vi "WhiteScreenTest_Startup.vi"() -> (0 "ErrorOut":errorcluster)   [LabVIEW 2018] (continued)
-inf, -inf, -inf, -inf, -inf, -inf, -inf, -inf, -inf, -inf, -inf, -inf, -inf, -inf, -inf, -inf, -inf, -inf, -inf, -inf, -inf, -inf, -inf, -inf, -inf, -inf, -inf, -inf, -inf, -inf, -inf, -inf, -inf, -inf, -inf, -inf, -inf, -inf, -inf, -inf, -inf, -inf, -inf, -inf, -inf, -inf, -inf, -inf, -inf, -inf, -inf, -inf, -inf, -inf, -inf, -inf, -inf, -inf, -inf, -inf, -inf, -inf, -inf, -inf, -inf, -inf, -inf, -inf, -inf, -inf, -inf, -inf, -inf, -inf, -inf, -inf, -inf, -inf, -inf, -inf, -inf, -inf, -inf, -inf, -inf, -inf, -inf, -inf, -inf, -inf, -inf, -inf, -inf, -inf, -inf, -inf, -inf, -inf, -inf, -inf, -inf, -inf, -inf, -inf, -inf, -inf, -inf, -inf, -inf, -inf, -inf, -inf, -inf, -inf, -inf, -inf, -inf, -inf, -inf, -inf, -inf, -inf, -inf, -inf, -inf, -inf, -inf, -inf, -inf, -inf, -inf, -inf, -inf, -inf, -inf, -inf, -inf, -inf, -inf, -inf, -inf, -inf, -inf, -inf, -inf, -inf, -inf, -inf, -inf, -inf, -inf, -inf, -inf, -inf, -inf, -inf, -inf, -inf, -inf, -inf, -inf, -inf, -inf, -inf, -inf, -inf, -inf, -inf, -inf, -inf, -inf, -inf, -inf, -inf, -inf, -inf, -inf, -inf, -inf, -inf, -inf, -inf, -inf, -inf, -inf, -inf, -inf, -inf, -inf, -inf, -inf, -inf, -inf, -inf, -inf, -inf, -inf, -inf, -inf, -inf, -inf, -inf, -inf, -inf, -inf, -inf, -inf, -inf, -inf, -inf, -inf, -inf, -inf, -inf, -inf, -inf, -inf, -inf, -inf, -inf, -inf, -inf, -inf, -inf, -inf, -inf, -inf, -inf, -inf, -inf, -inf, -inf, -inf, -inf, -inf, -inf, -inf, -inf, -inf, -inf, -inf, -inf, -inf, -inf, -inf, -inf, -inf, -inf, -inf, -inf, -inf, -inf, -inf, -inf, -inf, -inf, -inf, -inf, -inf, -inf, -inf, -inf, -inf, -inf, -inf, -inf, -inf, -inf, -inf, -inf, -inf, -inf, -inf, -inf, -inf, -inf, -inf, -inf, -inf, -inf, -inf, -inf, -inf, -inf, -inf, -inf, -inf, -inf, -inf, -inf, -inf, -inf, -inf, -inf, -inf, -inf, -inf, -inf, -inf, -inf, -inf, -inf, -inf, -inf, -inf, -inf, -inf, -inf, -inf, -inf, -inf, -inf, -inf, -inf, -inf, -inf, -inf, -inf, -inf, -inf, -inf, -inf, -inf, -inf, -inf, -inf, -inf, -inf, -inf, -inf, -inf, -inf, -inf, -inf, -inf, -inf, -inf, -inf, -inf, -inf, -inf, -inf, -inf, -inf, -inf, -inf, -inf, -inf, -inf, -inf, -inf, -inf, -inf, -inf, -inf, -inf, -inf, -inf, -inf, -inf, -inf, -inf, -inf, -inf, -inf, -inf, -inf, -inf, -inf, -inf, -inf, -inf, -inf, -inf, -inf, -inf, -inf, -inf, -inf, -inf, -inf, -inf, -inf, -inf, -inf, -inf, -inf, -inf, -inf, -inf, -inf, -inf, -inf, -inf, -inf, -inf, -inf, -inf, -inf, -inf, -inf, -inf, -inf, -inf, -inf, -inf, -inf, -inf, -inf, -inf, -inf, -inf, -inf, -inf, -inf, -inf, -inf, -inf, -inf, -inf, -inf, -inf, -inf, -inf, -inf, -inf, -inf, -inf, -inf, -inf, -inf, -inf, -inf, -inf, -inf, -inf, -inf, -inf, -inf, -inf, -inf, -inf, -inf, -inf, -inf, -inf, -inf, -inf, -inf, -inf, -inf, -inf, -inf, -inf, -inf, -inf, -inf, -inf, -inf, -inf, -inf, -inf, -inf, -inf, -inf, -inf, -inf, -inf, -inf, -inf, -inf, -inf, -inf, -inf, -inf, -inf, -inf, -inf, -inf, -inf, -inf, -inf, -inf, -inf, -inf, -inf, -inf, -inf, -inf, -inf, -inf, -inf, -inf, -inf, -inf, -inf, -inf, -inf, -inf, -inf, -inf, -inf, -inf, -inf, -inf, -inf, -inf, -inf, -inf, -inf, -inf, -inf, -inf, -inf, -inf, -inf, -inf, -inf, -inf, -inf, -inf, -inf, -inf, -inf, -inf, -inf, -inf, -inf, -inf, -inf, -inf, -inf, -inf, -inf, -inf, -inf, -inf, -inf, -inf, -inf, -inf, -inf, -inf, -inf, -inf, -inf, -inf, -inf, -inf, -inf, -inf, -inf, -inf, -inf, -inf, -inf, -inf, -inf, -inf, -inf, -inf, -inf, -inf, -inf, -inf, -inf, -inf, -inf, -inf, -inf, -inf, -inf, -inf, -inf, -inf, -inf, -inf, -inf, -inf, -inf, -inf, -inf, -inf, -inf, -inf, -inf, -inf, -inf, -inf, -inf, -inf, -inf, -inf, -inf, -inf, -inf, -inf, -inf, -inf, -inf, -inf, -inf, -inf, -inf, -inf, -inf, -inf, -inf, -inf, -inf, -inf, -inf, -inf, -inf, -inf, -inf, -inf, -inf, -inf, -inf, -inf, -inf, -inf, -inf, -inf, -inf, -inf, -inf, -inf, -inf, -inf, -inf, -inf, -inf, -inf, -inf, -inf, -inf, -inf, -inf, -inf, -inf, -inf, -inf, -inf, -inf, -inf, -inf, -inf, -inf, -inf, -inf, -inf, -inf, -inf, -inf, -inf, -inf, -inf, -inf, -inf, -inf, -inf, -inf, -inf, -inf, -inf, -inf, -inf, -inf, -inf, -inf, -inf, -inf, -inf, -inf, -inf, -inf, -inf, -inf, -inf, -inf, -inf, -inf, -inf, -inf, -inf, -inf, -inf, -inf, -inf, -inf, -inf, -inf, -inf, -inf, -inf, -inf, -inf, -inf, -inf, -inf, -inf, -inf, -inf, -inf, -inf, -inf, -inf, -inf, -inf, -inf, -inf, -inf, -inf, -inf, -inf, -inf, -inf, -inf, -inf, -inf, -inf, -inf, -inf, -inf, -inf, -inf, -inf, -inf, -inf, -inf, -inf, -inf, -inf, -inf, -inf, -inf, -inf, -inf, -inf, -inf, -inf, -inf, -inf, -inf, -inf, -inf, -inf, -inf, -inf, -inf, -inf, -inf, -inf, -inf, -inf, -inf, -inf, -inf, -inf, -inf, -inf, -inf, -inf, -inf, -inf, -inf]
  out "df (Hz)":dbl=15258.7890625
  in  "AutoScale Y Noise":bool caption="AutoScale Y"
  in  "AvgAvg":bool caption="Average over 1 minute"
  out "Power History 84 X":T13(graph)
  out "Power History 84 Co":T13(graph)
  out "Power History 72 X":T13(graph)
  out "Power History 72 Co":T13(graph)
  in  "NewValueWeighting":dbl=0.75 min=0.01 max=1.0 step=0.01
  out "Freq History 84 Co":cluster{dbl, dbl, dbl}(graph)
  out "Freq History 84 X":cluster{dbl, dbl, dbl}(graph)
  out "Freq History 72 X":cluster{dbl, dbl, dbl}(graph)
  out "Freq History 72 Co":cluster{dbl, dbl, dbl}(graph)
  out "Inclinometer Std Dev History":T14(graph)
  out "Inclinometer History":T14(graph)
  out "VoltageDisplay":T15={"AI0_Unused"=0.033825768742891164, "AI1_-5V"=0.03350358521901454, "AI2_+5V"=0.03414795226674084, "AI3_+6V"=-0.0003256849402108635, "AI4_+12V"=-0.0012922355206829907, "AI5_+15V"=-0.0012922355206829907, "AI6_+28V"=-0.020301063655153495, "Ai16_72GHz_CalPower"=-0.0022587861014084333, "Ai17_84GHz_CalPower"=-0.0038697037365145624, "Ai18_InclinometerAz"=-0.0038697037365145624, "Ai19_InclinometerEl"=-0.0038697037365145624, "Az_StdDev"=-0.0038697037365145624, "El_StdDev"=-0.0038697037365145624, "Ai20_BlowerPower"=-0.0038697037365145624} caption="Voltage" {"Ai20_BlowerPower" format="%#.2g"; "El_StdDev" format="%#.2g"; "Az_StdDev" format="%#.2g"; "Ai19_InclinometerEl" format="%#.2g"; "Ai18_InclinometerAz" format="%#.2g"; "Ai17_84GHz_CalPower" format="%#.4g"; "Ai16_72GHz_CalPower" format="%#.4g"; "AI6_+28V" format="%#.2g"; "AI5_+15V" format="%#.2g"; "AI4_+12V" format="%#.2g"; "AI3_+6V" format="%#.2g"; "AI2_+5V" format="%#.2g"; "AI1_-5V" format="%#.2g"; "AI0_Unused" format="%#.2g"}
  out "TCsDisplay":T16={"TC0_LP1_Hi"=25.446637506096643, "TC1_LP1_MidHi"=-67954.67080824148, "TC2_LP1_Mid"=-67954.0860092046, "TC3_LP1_LoMid"=-68014.21654976695, "TC4_LP1_Lo"=-68013.6313297234, "TC5_LP2_Hi"=-68014.21654976695, "TC6_LP2_MidHi"=-68058.43020070596, "TC7_LP2_Mid"=-68059.01573745323, "TC8_LP2_LoMid"=-67937.01745222262, "TC9_LP2_Lo"=-67937.60213056742, "TC10_HVAC_Cond_In"=-67937.01745222262, "TC11_HVAC_Cond_Out"=-68021.98391844248, "TC12_Gen_Exhaust"=-68021.39864348577, "TC13_Tamb_Interior"=-68021.39864348577} caption="Thermocouples" {"TC13_Tamb_Interior" format="%#.1f"; "TC12_Gen_Exhaust" format="%#.1f"; "TC11_HVAC_Cond_Out" format="%#.1f"; "TC10_HVAC_Cond_In" format="%#.1f"; "TC9_LP2_Lo" format="%#.1f"; "TC8_LP2_LoMid" format="%#.1f"; "TC7_LP2_Mid" format="%#.1f"; "TC6_LP2_MidHi" format="%#.1f"; "TC5_LP2_Hi" format="%#.1f"; "TC4_LP1_Lo" format="%#.1f"; "TC3_LP1_LoMid" format="%#.1f"; "TC2_LP1_Mid" format="%#.1f"; "TC1_LP1_MidHi" format="%#.1f"; "TC0_LP1_Hi" format="%#.1f"}
  out "84CoCalFrq":dbl format="%#.9f"
  out "MaxValue_Cal_84X":dbl format="%#.2g"
  out "84CoBeacFrq":dbl format="%#.9f"
  out "MaxValue_Cal_72X":dbl format="%#.2g"
  out "72CoCalFrq":dbl format="%#.9f"
  out "72CoBeacFrq":dbl format="%#.2f"
  out "ADAM-Noise":dbl format="%#.2g"
  out "ADAM-CalEncl":dbl format="%#.2g"
  out "ADAM-XPol":dbl format="%#.2g"
  out "ADAM-Co":dbl format="%#.2g"
  out "TE_Front":dbl format="%#.2g"
  out "TE_Bottom":dbl format="%#.2g"
  out "TE_Air":dbl format="%#.2g"
  out "InclEl":dbl format="%#.2g"
  out "InclAz":dbl format="%#.2g"
  out "MaxValue_Cal_84Co":dbl format="%#.2g"
  out "MaxValue_Cal_72Co":dbl format="%#.2g"
  out "+28":dbl format="%#.2g"
  out "+15":dbl format="%#.2g"
  out "+12":dbl format="%#.2g"
  out "+6":dbl format="%#.2g"
  out "+5":dbl format="%#.2g"
  out "-5V":dbl format="%#.2g"
  out "ConnextIntTemp":dbl format="%#.2g"
  in  "AlarmThresholds_OneChan":T17={"Enbl"=FALSE, "ErrsAndWarns"={2.256637168141593, 5.663716814159292, 7.168141592920354, 9.336283185840708}} {"ErrsAndWarns" scale=0.0..10.0}
  in  "AlarmSettings":T18={"TC13"={"Enbl"=FALSE, "ErrsAndWarns"={0.0, 5.663716814159292, 7.168141592920354, 8.584070796460177}}, "AI1"={"Enbl"=FALSE, "ErrsAndWarns"={0.0, 5.663716814159292, 7.168141592920354, 8.584070796460177}}, "AI2"={"Enbl"=FALSE, "ErrsAndWarns"={0.0, 5.663716814159292, 7.168141592920354, 8.584070796460177}}, "AI3"={"Enbl"=FALSE, "ErrsAndWarns"={0.0, 5.663716814159292, 7.168141592920354, 8.584070796460177}}, "AI4"={"Enbl"=FALSE, "ErrsAndWarns"={0.0, 5.663716814159292, 7.168141592920354, 8.584070796460177}}, "AI5"={"Enbl"=FALSE, "ErrsAndWarns"={0.0, 5.663716814159292, 7.168141592920354, 8.584070796460177}}, "AI6"={"Enbl"=FALSE, "ErrsAndWarns"={0.0, 5.663716814159292, 7.168141592920354, 8.584070796460177}}, "AI18"={"Enbl"=FALSE, "ErrsAndWarns"={0.0, 5.663716814159292, 7.168141592920354, 8.584070796460177}}, "AI19"={"Enbl"=FALSE, "ErrsAndWarns"={0.0, 5.663716814159292, 7.168141592920354, 8.584070796460177}}, "TE1"={"Enbl"=FALSE, "ErrsAndWarns"={0.0, 5.663716814159292, 7.168141592920354, 8.584070796460177}}, "TE2"={"Enbl"=TRUE, "ErrsAndWarns"={0.0, 5.663716814159292, 7.168141592920354, 8.584070796460177}}, "TE3"={"Enbl"=FALSE, "ErrsAndWarns"={0.0, 5.663716814159292, 7.168141592920354, 8.584070796460177}}, "ADAM1"={"Enbl"=FALSE, "ErrsAndWarns"={0.0, 5.663716814159292, 7.168141592920354, 8.584070796460177}}, "ADAM2"={"Enbl"=FALSE, "ErrsAndWarns"={0.0, 5.663716814159292, 7.168141592920354, 8.584070796460177}}, "ADAM3"={"Enbl"=FALSE, "ErrsAndWarns"={0.0, 5.663716814159292, 7.168141592920354, 8.584070796460177}}, "ADAM4"={"Enbl"=FALSE, "ErrsAndWarns"={0.0, 5.663716814159292, 7.168141592920354, 8.584070796460177}}, "72CoBeacFreq"={"Enbl"=FALSE, "ErrsAndWarns"={0.0, 5.663716814159292, 7.168141592920354, 8.584070796460177}}, "72CoCalFreq"={"Enbl"=FALSE, "ErrsAndWarns"={0.0, 5.663716814159292, 7.168141592920354, 8.584070796460177}}, "84CoBeacFreq"={"Enbl"=FALSE, "ErrsAndWarns"={0.0, 5.663716814159292, 7.168141592920354, 8.584070796460177}}, "84CoCalFreq"={"Enbl"=FALSE, "ErrsAndWarns"={0.0, 5.663716814159292, 7.168141592920354, 8.584070796460177}}, "72Co_CalTonePwr"={"Enbl"=FALSE, "ErrsAndWarns"={-110.0, -90.0, -65.0, -60.0}}, "72X_CalTonePwr"={"Enbl"=FALSE, "ErrsAndWarns"={0.0, 5.663716814159292, 7.168141592920354, 8.584070796460177}}, "84Co_CalTonePwr"={"Enbl"=FALSE, "ErrsAndWarns"={0.0, 5.663716814159292, 7.168141592920354, 8.584070796460177}}, "84X_CalTonePwr"={"Enbl"=FALSE, "ErrsAndWarns"={0.0, 5.663716814159292, 7.168141592920354, 8.584070796460177}}} {"84X_CalTonePwr"."ErrsAndWarns" scale=-120.0..-55.0; "72X_CalTonePwr"."ErrsAndWarns" scale=-120.0..-55.0; "84Co_CalTonePwr"."ErrsAndWarns" scale=-120.0..-55.0; "72Co_CalTonePwr"."ErrsAndWarns" scale=-120.0..-55.0; "84CoCalFreq"."ErrsAndWarns" scale=24.9..25.1; "84CoBeacFreq"."ErrsAndWarns" scale=25.3..25.8; "72CoCalFreq"."ErrsAndWarns" scale=24.9..25.1; "72CoBeacFreq"."ErrsAndWarns" scale=25.4..25.8; "ADAM4"."ErrsAndWarns" scale=30.0..52.0; "ADAM3"."ErrsAndWarns" scale=30.0..52.0; "ADAM2"."ErrsAndWarns" scale=30.0..52.0; "ADAM1"."ErrsAndWarns" scale=30.0..52.0; "TE3"."ErrsAndWarns" scale=30.0..52.0; "TE2"."ErrsAndWarns" scale=30.0..52.0; "TE1"."ErrsAndWarns" scale=20.0..52.0; "AI19"."ErrsAndWarns" scale=0.0..6.0; "AI18"."ErrsAndWarns" scale=0.0..8.0; "AI6"."ErrsAndWarns" scale=0.0..35.0; "AI5"."ErrsAndWarns" scale=0.0..20.0; "AI4"."ErrsAndWarns" scale=0.0..15.0; "AI3"."ErrsAndWarns" scale=0.0..10.0; "AI2"."ErrsAndWarns" scale=0.0..10.0; "TC13"."ErrsAndWarns" scale=0.0..40.0}
  out "Elapsed_SNR_Timer":dbl caption="Elapsed SNR Timer"
  in  "Trouble Shooting Tabs":T19(tab)
  out "Q Probes":T20
  out "Probe 21":fxp<+/-,24,5>=-4.57763671875e-05
  out "Probe 22":fxp<+/-,54,35>=-15871.999969482422
  out "Probe 23":fxp<+/-,54,1>=-7.629394517039145e-06
  out "Probe 24":fxp<+/-,16,1>
  out "I Probes":T20
  out "Probe 3":fxp<+/-,39,24>=-0.003662109375
  out "Probe 1":i16=-27
  out "Probe 2":fxp<+/-,16,16>
  out "Probe 5":fxp<+/-,16,2>
  out "Probe 7":fxp<+/-,18,1>
  out "ReceiverTimed Out":bool
  out "NoiseFloorFIFOTimeOut":bool
  out "Probe Offsetd":fxp<+/-,16,16>
  in  "Target to Probe":T21=enum."4"
  in  "Time Domain Tabs":T22(tab)
  out "TimeDomainCal":ext[](graph)
  out "TimeDomainBeac":ext[](graph)
  out "TimeDomainCal 2":ext[](graph)
  out "TimeDomainBeacon 2":ext[](graph)
  out "TimeDomainCal 3":ext[](graph)
  out "TimeDomain Beac 3":ext[](graph)
  out "InPhase Spect":dbl[](graph)
  out "QuadratureSpect":dbl[](graph)
  out "TimeDomainCal 4":ext[](graph)
  out "TimeDomainBeacon 4":ext[](graph)
  out "Memory Used":dbl(graph)=797012.0
  out "CalShift 2":dbl=24999500.0 format="%#_10g"
  out "BeaconShift 2":dbl=26246000.0 format="%#_10g"
  out "BeaconShift":dbl=26246000.0 format="%#_10g"
  out "CalShift":dbl=24999500.0 format="%#_10g"
  out "FAM Initialized?":bool=TRUE
  out "Memory Used By LV (KB)":dbl=797012.0
  out "BeaconShift 4":dbl=26244800.0 format="%#_10g"
  out "BeaconShift 3":dbl=26246000.0 format="%#_10g"
  out "CalShift 3":dbl=24999500.0 format="%#_10g"
  out "CalShift 4":dbl=24998000.0 format="%#_10g"
  in  "MemoryPlotRate":dbl=30.0 format="%#_13g"
  out "SPVSR_Count":i32
  out "SPVSR_Queue":i32
  out "FP_Count":i32
  out "# in FP queue":i32
  out "PhaseCount 1":u64
  out "PhaseCount 2":u64
  out "PhaseCount 3":u64
  out "PhaseCount 4":u64
  out "X I_Index":ext[](array[numeric])
  out "72 Co Beac Q":ext[](graph)
  out "72 Co Beac I":ext[](graph)
  out "Co I_Index":ext[](array[numeric])
  in  "Exit":bool
  in  "Stop":bool
  # "Ugh5"
  # "Copyright © 2020 Epimedia, Inc. All Rights Reserved.\n\nThe Epimedia Application Library is Copyright © 2009-2020 Epimedia, Inc. \nAll Rights Reserved. Used under license."
  # "Angle_out = [(V_reading – Vmin) / Vmax ) * (Angle_max - Angle_min) + Angle_min + Angle_offset ] * (-1 if pos_neg toggle switch is on)\n\nThe default (equivalent to current equation) values would be\nVmin = 0\nVmax = 4.5\nAngle_min = -90\nAngle_range = Angle_max-Angle_min\nAngle_max = 90\nAngle_offset = 0\nPos_neg = off"
  # "72 Cross Tracking Frequency is linked to 72 Co"
  # "84 Cross Tracking Frequency is linked to 84 Co"
  # "72 Co"
  # "84 Co"
  # "72 GHz"
  # "84 GHz"
  # "Enable/disable"
  # "The digital readouts display the same errors and \nwarnings with more precision."
  # "Low Error"
  # "Low Warning"
  # "High Warning"
  # "High Error"
  # "seconds"
  # "I Probes"
  # "Q Probes"
  # "-1 to 0.999, d:7.629e-6"
  # "Shifted"
  # "I16"
  # "-1 to 1, d:1.92e-7"
  # "From digitizer"
  # "Filtered Step 4"
  # "-3.27e4 to 3.27e4, d:1"
  # "-1 to 1, d:1.92e-7"
  # "To FXP"
  # "Scaled and reduced data size"
  # "-3.27e4 to 3.27e4, d:1"
  # "-1 to 1, d:1.92e-7"
  # "Filtered Step 5"
  # "-6.55e4 to 6.55e4, d:3.05e-5"
  # "-8.39e6 to 8.39e6, d:1.19e-7"
  # "Scaled"
  # "Scaled after Step 5"
  # "XXX"
  # "-2 to 2, d:2.38e-7"
  # "-2 to 1.999, d:6.10e-5"
  # "Filtered Step 6"
  # "Filtered stage A"
  # "-1.677e7 to 1.677e7, d:2.38e-7"
  # "Scaled after Step 6"
  # "XXX"
  # "-2.62e5 to 2.62e5, d:6.10e-5"
  # "Scaled (Step 1 Scale)"
  # "-1 to 1, d:1.82e-12"
  # "Filtered Step 7"
  # "-8.39e6 to 8.39e6, d:1.82e-12"
  # "Filtered after Step 7"
  # "XXX"
  # "-8.39e6 to 8.39e6, d:1.82e-12"
  # "Sent to host\nIdentical to 18"
  # "Noise Floor"
  # "-4 to 4"
  # "-3.35e7 to 3.35e7, d:4.7e-7"
  # "-1 to 1, d:1.4e-14"
  # "-1 to .99, d:3.05e-5"
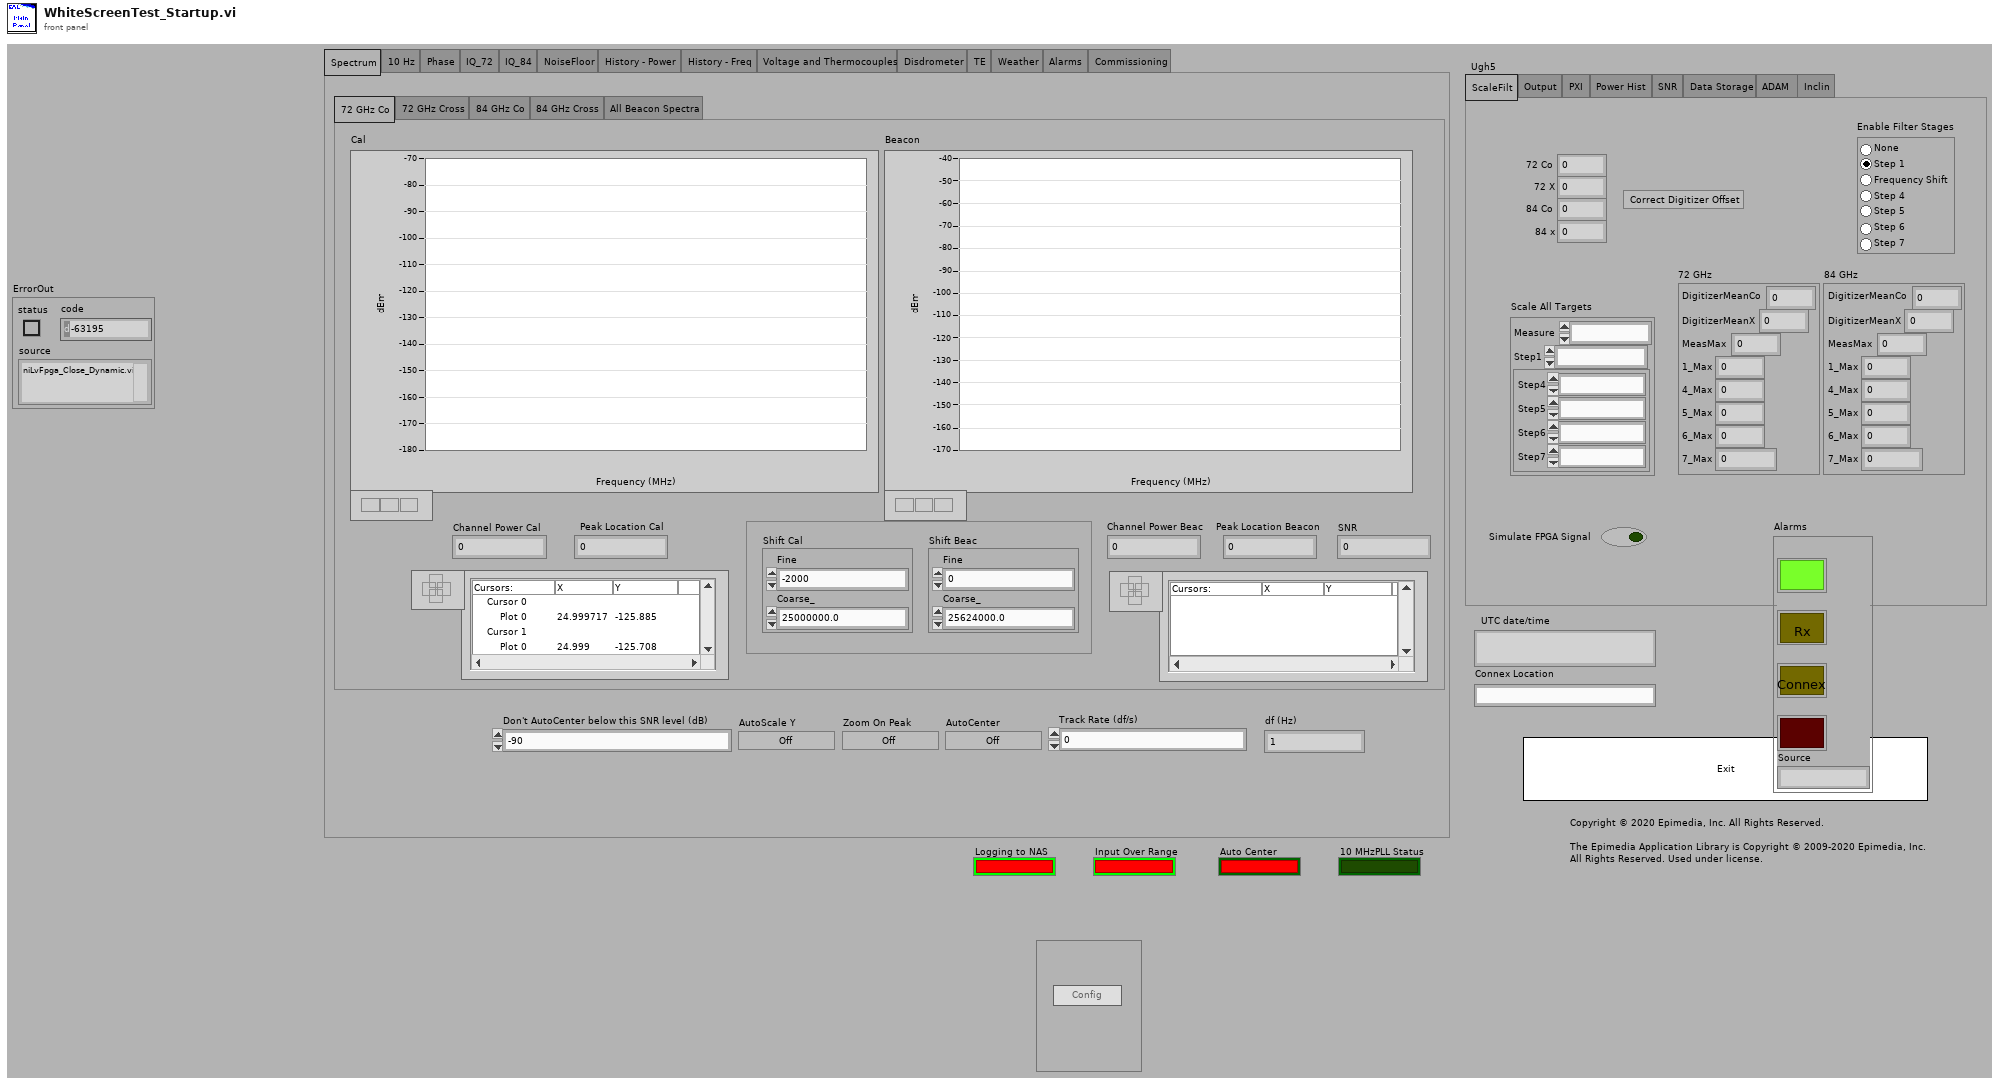
[diagram p1: front panel]
types:
  T1 = typedef "DigOutClust.ctl" = cluster{"Green":bool, "Rx_Yell":bool, "Cx_Yell":bool, "Red":bool, "Source":string}
  T2 = enum32{"ScaleFilt", "Output", "PXI", "Power Hist", "SNR", "Data Storage", "ADAM", "Inclin"}
  T3 = typedef "SaturationMonitor.ctl" = cluster{"MeasMean0":dbl, "MeasMean1":dbl, "MeasMax":dbl, "1_Max":dbl, "4_Max":dbl, "5_Max":dbl, "6_Max":dbl, "7_Max":dbl}
  T4 = typedef "ScaleTargetClust.ctl" = cluster{"Measure":fxp<+/-,16,1>, "Step1":fxp<+/-,17,17>, "Scale":T5}
  T5 = typedef "FPGA_Scale.ctl" = cluster{"Step4":fxp<+/-,23,23>, "Step5":fxp<+/-,23,23>, "Step6":fxp<+/-,23,23>, "Step7":fxp<+/-,23,23>}
  T6 = typedef "FilterEnableRadio.ctl" = enum32{"None", "Step 1", "Frequency Shift", "Step 4", "Step 5", "Step 6", "Step 7"}
  T7 = cluster{"Cal Smooth":dbl, "Beac Smooth":dbl, "Cal Smooth":dbl, "Beac Smooth":dbl, "Cal Smooth":dbl, "Beac Smooth":dbl, "Cal Smooth":dbl, "Beac Smooth":dbl}
  T8 = typedef "Inclinometer_User_Cfg.ctl" = cluster{"Vmin":dbl, "Vmax":dbl, "Angle_min":dbl, "Angle_max":dbl, "Offset":dbl, "Pos_Neg":bool}
  T9 = enum32{"Spectrum", "10 Hz", "Phase", "IQ_72", "IQ_84", "NoiseFloor", "History - Power", "History - Freq", "Voltage and Thermocouples", "Disdrometer", "TE", "Weather", "Alarms", "Commissioning"}
  T10 = enum32{"72 GHz Co", "72 GHz Cross", "84 GHz Co", "84 GHz Cross", "All Beacon Spectra"}
  T11 = typedef "FreqShift.ctl" = cluster{"Fine":dbl, "Coarse_":dbl}
  T12 = enum32{"72 GHz Co", "72 GHz Cross", "84 GHz Co", "84 GHz Cross"}
  T13 = cluster{"Cal":dbl, "Cal Smooth":dbl, "Beac":dbl, "Beac Smooth":dbl, "NoiseFloorSum":dbl, "NoiseFloorSum Smooth":dbl}
  T14 = cluster{"Ai18_InclinometerAz":dbl, "Ai19_InclinometerEl":dbl}
  T15 = typedef "Voltage_Display_Clust.ctl" = cluster{"AI0_Unused":dbl, "AI1_-5V":dbl, "AI2_+5V":dbl, "AI3_+6V":dbl, "AI4_+12V":dbl, "AI5_+15V":dbl, "AI6_+28V":dbl, "Ai16_72GHz_CalPower":dbl, "Ai17_84GHz_CalPower":dbl, "Ai18_InclinometerAz":dbl, "Ai19_InclinometerEl":dbl, "Az_StdDev":dbl, "El_StdDev":dbl, "Ai20_BlowerPower":dbl}
  T16 = typedef "TC_Display_Clust.ctl" = cluster{"TC0_LP1_Hi":dbl, "TC1_LP1_MidHi":dbl, "TC2_LP1_Mid":dbl, "TC3_LP1_LoMid":dbl, "TC4_LP1_Lo":dbl, "TC5_LP2_Hi":dbl, "TC6_LP2_MidHi":dbl, "TC7_LP2_Mid":dbl, "TC8_LP2_LoMid":dbl, "TC9_LP2_Lo":dbl, "TC10_HVAC_Cond_In":dbl, "TC11_HVAC_Cond_Out":dbl, "TC12_Gen_Exhaust":dbl, "TC13_Tamb_Interior":dbl}
  T17 = typedef "AlarmThresh_OneChan.ctl" = cluster{"Enbl":bool, "ErrsAndWarns":cluster{dbl, dbl, dbl, dbl}}
  T18 = typedef "AlarmSettingsClust.ctl" = cluster{"TC13":T17, "AI1":T17, "AI2":T17, "AI3":T17, "AI4":T17, "AI5":T17, "AI6":T17, "AI18":T17, "AI19":T17, "TE1":T17, "TE2":T17, "TE3":T17, "ADAM1":T17, "ADAM2":T17, "ADAM3":T17, "ADAM4":T17, "72CoBeacFreq":T17, "72CoCalFreq":T17, "84CoBeacFreq":T17, "84CoCalFreq":T17, "72Co_CalTonePwr":T17, "72X_CalTonePwr":T17, "84Co_CalTonePwr":T17, "84X_CalTonePwr":T17}
  T19 = enum32{"FPGA Probes", "Time Domain", "Win Probes", "DeltaPhaseTest"}
  T20 = cluster{"Probe 8":fxp<+/-,18,1>, "Probe 9":fxp<+/-,24,1>, "Probe 10":fxp<+/-,24,1>, "Probe 11":fxp<+/-,24,1>, "Probe 12":fxp<+/-,47,24>, "Probe 13":fxp<+/-,24,1>, "Probe 14":fxp<+/-,25,2>, "Probe 15":fxp<+/-,48,25>, "Probe 16":fxp<+/-,24,1>, "Probe 17":fxp<+/-,25,2>, "Probe 18":fxp<+/-,48,25>, "Probe 19":fxp<+/-,24,1>, "Probe20":fxp<+/-,24,1>}
  T21 = typedef "TargetNumber.ctl" = enum16{"1", "2", "3", "4"}
  T22 = enum32{"Target 1", "Target 2", "Target 3", "Complex Spectra", "Target 4"}
  T23 = typedef "10Hz_Loop_Enum.ctl" = enum16{"10Hz_Init", "10Hz_Cfg", "10Hz_NewData", "10Hz_Write", "10Hz_Stop"}
  T24 = typedef "FP_Loop_Clust.ctl" = cluster{"Alarms":T1, "Spectrum 1":dbl[], "Spectrum 2":dbl[], "Spectrum 3":dbl[], "Spectrum 4":dbl[], "HistoryWeighting":dbl, "NoiseFloorSums":T25, "PwrHist":T26}
  T25 = typedef "NoiseFLoorSums.ctl" = cluster{"1":dbl, "2":dbl, "3":dbl, "4":dbl}
  T26 = typedef "PowerHistory_All.ctl" = cluster{"72Co":cluster{"Cal":dbl, "Cal Smooth":dbl, "Beac":dbl, "Beac Smooth":dbl, "NoiseFloorSum":dbl, "NoiseFloorSum Smooth":dbl}, "72X":cluster{"Cal":dbl, "Cal Smooth":dbl, "Beac":dbl, "Beac Smooth":dbl, "NoiseFloorSum":dbl, "NoiseFloorSum Smooth":dbl}, "84Co":cluster{"Cal":dbl, "Cal Smooth":dbl, "Beac":dbl, "Beac Smooth":dbl, "NoiseFloorSum":dbl, "NoiseFloorSum Smooth":dbl}, "84X":cluster{"Cal":dbl, "Cal Smooth":dbl, "Beac":dbl, "Beac Smooth":dbl, "NoiseFloorSum":dbl, "NoiseFloorSum Smooth":dbl}}
  T27 = typedef "HWQueueElements.ctl" = enum16{"HW_Init", "HW_UpdtCfg", "HW_Start", "HW_Pause", "HW_Run", "HW_Cls", "HW_Exit"}
  T28 = typedef "FP_Loop_Enum.ctl" = enum16{"FP_Init", "FP_Scale", "FP_Tone", "FP_Noise", "FP_Probes", "FP_PXI", "FP_AI", "FP_TC", "FP_PWR_Hist", "FP_Alarm", "FP_Exit"}
  T29 = typedef "DigiLoopEnum.ctl" = enum16{"Dig_Init", "Digi_Write", "Digi_Exit"}
  T30 = typedef "LogLoopEnum.ctl" = enum16{"Log_Init", "Log_Config", "Log_CfgAlarm", "Log_TimeDomain", "Log_Tone", "Log_NoiseTrace", "Log_NoiseSum", "Log_DO", "Log_AI", "Log_TC", "Log_Disdrom", "Log_Weather", "Log_TE", "Log_ADAM", "Log_UPS", "Log_ChkTime", "Log_Alarm", "Log_Write", "Log_Exit"}
  T31 = typedef "NoiseQueueElements.ctl" = enum16{"Noise_Startup", "Noise_Init", "Noise_Macro", "Noise_Config", "Noise_NewData", "Noise_Transform", "Noise_SumdTrace", "Noise_Send", "Noise_Probes", "Noise_Exit"}
  T32 = typedef "MasterCluster.ctl" = cluster{"Admin":T33, "RTConfig":T35, "SMS":T36, "FPGA":T37, "Config":T38, "Stat":T44, "Alarm":T18}
  T33 = typedef "AdminCluster.ctl" = cluster{"Lvl":T34, "Pwd":string}
  T34 = typedef "UserLevelEnum.ctl" = enum16{"Admin", "Operator"}
  T35 = typedef "RT_Config.ctl" = cluster{"Arm":bool, "Number":dbl, "String":string}
  T36 = typedef "SMSDataCluster.ctl" = cluster{"Enbl?":bool, "Addr":string[]}
  T37 = typedef "FPGA_Config_Clust.ctl" = cluster{"Target":T21, "Channel":T21, "Ref1":refnum<k20>, "Ref2":refnum<k20>}
  T38 = typedef "Config_Clust.ctl" = cluster{"UsrCfg":T39, "FP_User":T41}
  T39 = typedef "UserConfig.ctl" = cluster{"Paths":T40, "SampleRate":dbl}
  T40 = typedef "PathsCluster.ctl" = cluster{"CfgFile":path, "LogFolder":path, "LogFile":path, "NAS path":path, "ThreshFile":path, "RedunFolder":path}
  T41 = typedef "FrontPanel_UserConfig.ctl" = cluster{"#NoiseSums":u32, "Max_df":u32, "AvgAvg":bool, "#Avg":u16, "AutoCenter":bool, "Inclin":T8, "1":T42, "2":T42, "3":T42, "4":T42, "Target to Probe":T21, "SNR_Thresh":dbl, "Paths":T40, "Connex_Location":string, "SimulateFPGA":bool}
  T42 = typedef "FP_UserTargetConfig.ctl" = cluster{"Cal_":T11, "Beac":T11, "Scale":T5, "Offset":fxp<+/-,16,16>, "Scale_Noise":fxp<+/-,30,30>, "Scale_Step1":fxp<+/-,17,17>, "Scale_In_RT":ext, "ScaleMeas":fxp<+/-,16,1>, "FreqsToRemove":i32[], "Width":i32[], "ScaleMeasEnum":T43, "FilterEnab":T6}
  T43 = typedef "ScaleMeasure.ctl" = enum16{"1", "10", "50", "42"}
  T44 = typedef "SystemStatusCluster.ctl" = cluster{"SysState":T45, "TrackRate":bool, "AutoCentr":bool}
  T45 = typedef "SystemStateEnum.ctl" = enum16{"Init", "Idle", "Running", "System Fault", "System Error", "Exit"}
  T46 = typedef "DataQueueElements.ctl" = enum16{"Data_Init", "Data_Config", "Data_AddData", "Data_FreqShift", "Data_FPGA_Write", "Data_Transform", "Data_Send", "Data_Exit"}
  T47 = typedef "MainQueueElements.ctl" = enum16{"Spvsr_InitQ", "Spvsr_RfrshPnl", "Spvsr_InitSW", "Spvsr_InitCtrls", "Spvsr_Cursors", "Spvsr_StrtHWLp", "Spvsr_Stop", "Spvsr_NewData", "Spvsr_ScaleGraphs", "Spvsr_Error", "Spvsr_About", "Spvsr_Config", "Spvsr_FPConfig", "Spvsr_AlarmCfg", "Spvsr_DigitzOffs", "FP_AO_ctrl", "Spvsr_RestartWarn", "Spvsr_AutoCenter", "Spvsr_TrackRate", "Spvsr_ChkTime", "Spvsr_Admin", "Spvsr_Exit"}
  T48 = typedef "HDF5_10HzRefs.ctl" = cluster{"72Co_dset":T49, "84Co_dset":T49, "FileRef":T49}
  T49 = typedef "hid_t.ctl" = i32
  T50 = typedef "AI_Type_Enum.ctl" = enum16{"AI", "TC"}
  T51 = typedef "MainQueueElements.ctl" = enum16{"Spvsr_InitQ", "Spvsr_RfrshPnl", "Spvsr_InitSW", "Spvsr_InitCtrls", "Spvsr_Cursors", "Spvsr_StrtHWLp", "Spvsr_Stop", "Spvsr_NewData", "Spvsr_DigiOut", "Spvsr_ScaleGraphs", "Spvsr_Error", "Spvsr_About", "Spvsr_Config", "Spvsr_FPConfig", "Spvsr_AlarmCfg", "Spvsr_DigitzOffs", "FP_AO_ctrl", "Spvsr_RestartWarn", "Spvsr_AutoCenter", "Spvsr_TrackRate", "Spvsr_ChkTime", "Spvsr_Admin", "Spvsr_Exit"}
  T52 = enum8{"Enabled", "Disabled", "Disabled and Grayed Out"}
  T53 = typedef "AI_Loop_Enum.ctl" = enum16{"AI_Init", "AI_Config", "AI_Alarm", "AI_Read", "AI_ChkTime", "AI_Exit"}
  T54 = typedef "LVCursorListTypeDef.ctl" = cluster{"Name":string, "Color":u32, "Style":u8, "Point Style":u8, "Name Visible":bool, "Allow Drag":bool, "Cursor Mode":u32, "Plot":i32, "Index":i32, "Position":cluster{"X":dbl, "Y":dbl}, "X Scale":u32, "Y Scale":u32, "Watch Plots":i32[], "Watch All Plots":bool, "Plot Area":i32, "Label Offset":cluster{"X":dbl, "Y":dbl}}[]
  T55 = typedef "AO_Loop_Enum.ctl" = enum16{"AO_Init", "AO_Write", "AO_Exit"}
  T56 = typedef "TargetToneData.ctl" = cluster{"Cal":T57, "Beac":T57, "Time":timestamp[], "Saturat":T3}
  T57 = typedef "ChannelToneData.ctl" = cluster{"Shift_":dbl, "Peak_ToFPGA":dbl, "MaxValue":dbl, "MaxIndex":i32, "Tone":T58, "TimeDomainI":ext[], "TimeDomainQ":ext[], "PwrSpectrum":dbl[], "RunningAvgFreq":dbl, "ISpectPos":dbl[], "ISpectNeg":dbl[], "QSpectPos":dbl[], "QSpectNeg":dbl[], "10Hz_PwrSpectr":dbl[][], "SNR":dbl, "AliasWarn":bool, "10Hz_Peak":dbl[], "ISpect+-":dbl[], "QSpect+-":dbl[], "TimeStamp":timestamp, "I_Index":ext[], "Q_Index":ext[], "10MHz":bool}
  T58 = typedef "ToneInfoClust.ctl" = cluster{"PkLocTrak":dbl, "PkLocDisp":dbl, "df_":dbl, "ZoomPwr":dbl[], "Phase":dbl, "PhaseOld":dbl, "AboveThresh?":bool, "MaxI":dbl, "MaxQ":dbl, "median":dbl, "ISpect":dbl[], "QSpect":dbl[], "DeltaPhase":dbl}
  T59 = typedef "NoiseFloorData.ctl" = cluster{"df":dbl, "AvgAvgSpectrum":dbl[], "FFT_Index":i32[], "Avg'd":dbl[], "Sum":dbl, "SumdSpectrum":dbl[], "SumCount":u32}
  T60 = typedef "FPGA_Probes.ctl" = cluster{"Probe 1":i16, "Probe 2":fxp<+/-,16,16>, "Probe 3":fxp<+/-,39,24>, "Probe 4":fxp<+/-,39,24>, "Probe 5":fxp<+/-,16,2>, "Probe 6":fxp<+/-,33,19>, "Probe 7":fxp<+/-,18,1>, "Probe 7_1":fxp<+/-,18,1>, "IProbe":cluster{"Probe 8":fxp<+/-,18,1>, "Probe 9":fxp<+/-,24,1>, "Probe 10":fxp<+/-,24,1>, "Probe 11":fxp<+/-,24,1>, "Probe 12":fxp<+/-,47,24>, "Probe 13":fxp<+/-,24,1>, "Probe 14":fxp<+/-,25,2>, "Probe 15":fxp<+/-,48,25>, "Probe 16":fxp<+/-,24,1>, "Probe 17":fxp<+/-,25,2>, "Probe 18":fxp<+/-,48,25>, "Probe 19":fxp<+/-,24,1>, "Probe20":fxp<+/-,24,1>}, "Probe 21":fxp<+/-,24,5>, "Probe 22":fxp<+/-,54,35>, "Probe 23":fxp<+/-,54,1>, "Probe 24":fxp<+/-,16,1>, "Probe Offsetd":fxp<+/-,16,16>, "CalShiftProbe":fxp<+/-,48,0>, "QProbe":cluster{"Probe 8":fxp<+/-,18,1>, "Probe 9":fxp<+/-,24,1>, "Probe 10":fxp<+/-,24,1>, "Probe 11":fxp<+/-,24,1>, "Probe 12":fxp<+/-,47,24>, "Probe 13":fxp<+/-,24,1>, "Probe 14":fxp<+/-,25,2>, "Probe 15":fxp<+/-,48,25>, "Probe 16":fxp<+/-,24,1>, "Probe 17":fxp<+/-,25,2>, "Probe 18":fxp<+/-,48,25>, "Probe 19":fxp<+/-,24,1>, "Probe20":fxp<+/-,24,1>}, "AI_Over":bool, "10MHzLocked":bool}
  T61 = typedef "PXI_Health.ctl" = cluster{"Temperatures":string[][], "Fans":string[][], "Voltages":string[][]}
  T62 = typedef "All_AI_Error_and_Data.ctl" = cluster{"AI":T63, "AllErrorStatus":T64}
  T63 = typedef "AI_Clust.ctl" = cluster{"TimeString":string, "Time Stamp":dbl, "AI0_Unused":dbl, "AI1_-5V":dbl, "AI2_+5V":dbl, "AI3_+6V":dbl, "AI4_+12V":dbl, "AI5_+15V":dbl, "AI6_+28V":dbl, "AI7_Unused":dbl, "Ai16_72GHz_CalPower":dbl, "Ai17_84GHz_CalPower":dbl, "Ai18_InclinAz":dbl, "Ai19_InclinEl":dbl, "Ai20_BlowerPwr":dbl, "Ai21_Unused":dbl, "Ai22_Unused":dbl, "Ai23_Unused":dbl, "InclinA_StdDev":dbl, "InclinB_StdDev":dbl, "InclinAz_Unfilt":dbl, "InclinEl_Unfilt":dbl}
  T64 = typedef "All_AI_Error_Status.ctl" = cluster{"AI 0":T65, "AI 1":T65, "AI 2":T65, "AI 3":T65, "AI 4":T65, "AI 5":T65, "AI 6":T65, "AI 7":T65, "AI 16":T65, "AI 17":T65, "AI 18":T65, "AI 19":T65, "AI 20":T65, "AI 21":T65, "AI 22":T65, "AI 23":T65}
  T65 = typedef "ErrorStatus.ctl" = cluster{"RX?":bool, "Warn":bool, "Error":bool, "Enabl":bool, "Source":string}
  T66 = typedef "All_TC_Error_and_Data.ctl" = cluster{"TCData":T67, "All_TC_ErrorStatus":T68}
  T67 = typedef "TC_Data_Structure.ctl" = cluster{"TimeStamp":dbl, "TimeString":string, "TC0_LP1_Hi":dbl, "TC1_LP1_MidHi":dbl, "TC2_LP1_Mid":dbl, "TC3_LP1_LoMid":dbl, "TC4_LP1_Lo":dbl, "TC5_LP2_Hi":dbl, "TC6_LP2_MidHi":dbl, "TC7_LP2_Mid":dbl, "TC8_LP2_LoMid":dbl, "TC9_LP2_Lo":dbl, "TC10_HVAC_Cond_In":dbl, "TC11_HVAC_Cond_Out":dbl, "TC12_Gen_Exhaust":dbl, "TC13_Unused":dbl, "TC14_Unused":dbl, "TC15_Unused":dbl, "TC16_Unused":dbl, "TC17_Unused":dbl, "TC18_Unused":dbl, "TC19_Unused":dbl, "TC20_Unused":dbl, "TC21_Unused":dbl, "TC22_Unused":dbl, "TC23_Unused":dbl, "TC24_Unused":dbl, "TC25_Unused":dbl, "TC26_Unused":dbl, "TC27_Unused":dbl, "TC28_Unused":dbl, "TC29_Unused":dbl, "TC30_Unused":dbl, "TC31_Unused":dbl}
  T68 = typedef "All_TC_Error_Status.ctl" = cluster{"TC 0":T65, "TC 1":T65, "TC 2":T65, "TC 3":T65, "TC 4":T65, "TC 5":T65, "TC 6":T65, "TC 7":T65, "TC 8":T65, "TC 9":T65, "TC 10":T65, "TC 11":T65, "TC 12":T65, "TC 13":T65, "TC 14":T65, "TC 15":T65, "TC 16":T65, "TC 17":T65, "TC 18":T65, "TC 19":T65, "TC 20":T65}
  T69 = typedef "AlarmDisplay.ctl" = cluster{"Alarms":T1, "SerialMeas":T70, "AllAlarms":T65[], "Elapsed_SNR_Timer":dbl, "Saturation":T71}
  T70 = typedef "SerialMeasurements_Clust.ctl" = cluster{"TE_Air":dbl, "TE_Bottom":dbl, "TE_Front":dbl, "ADAM-Co":dbl, "ADAM-XPol":dbl, "ADAM-CalEncl":dbl, "ADAM-Noise":dbl}
  T71 = typedef "Saturation_Status_Clust.ctl" = cluster{"84":bool[], "72":bool[]}
  T72 = cluster{"Cal":dbl, "Cal Smooth":dbl, "Beac":dbl, "Beac Smooth":dbl, "NoiseFloorSum":dbl, "NoiseFloorSum Smooth":dbl}[]
  T73 = enum16{"Always On", "Always Off", "Off While Running"}
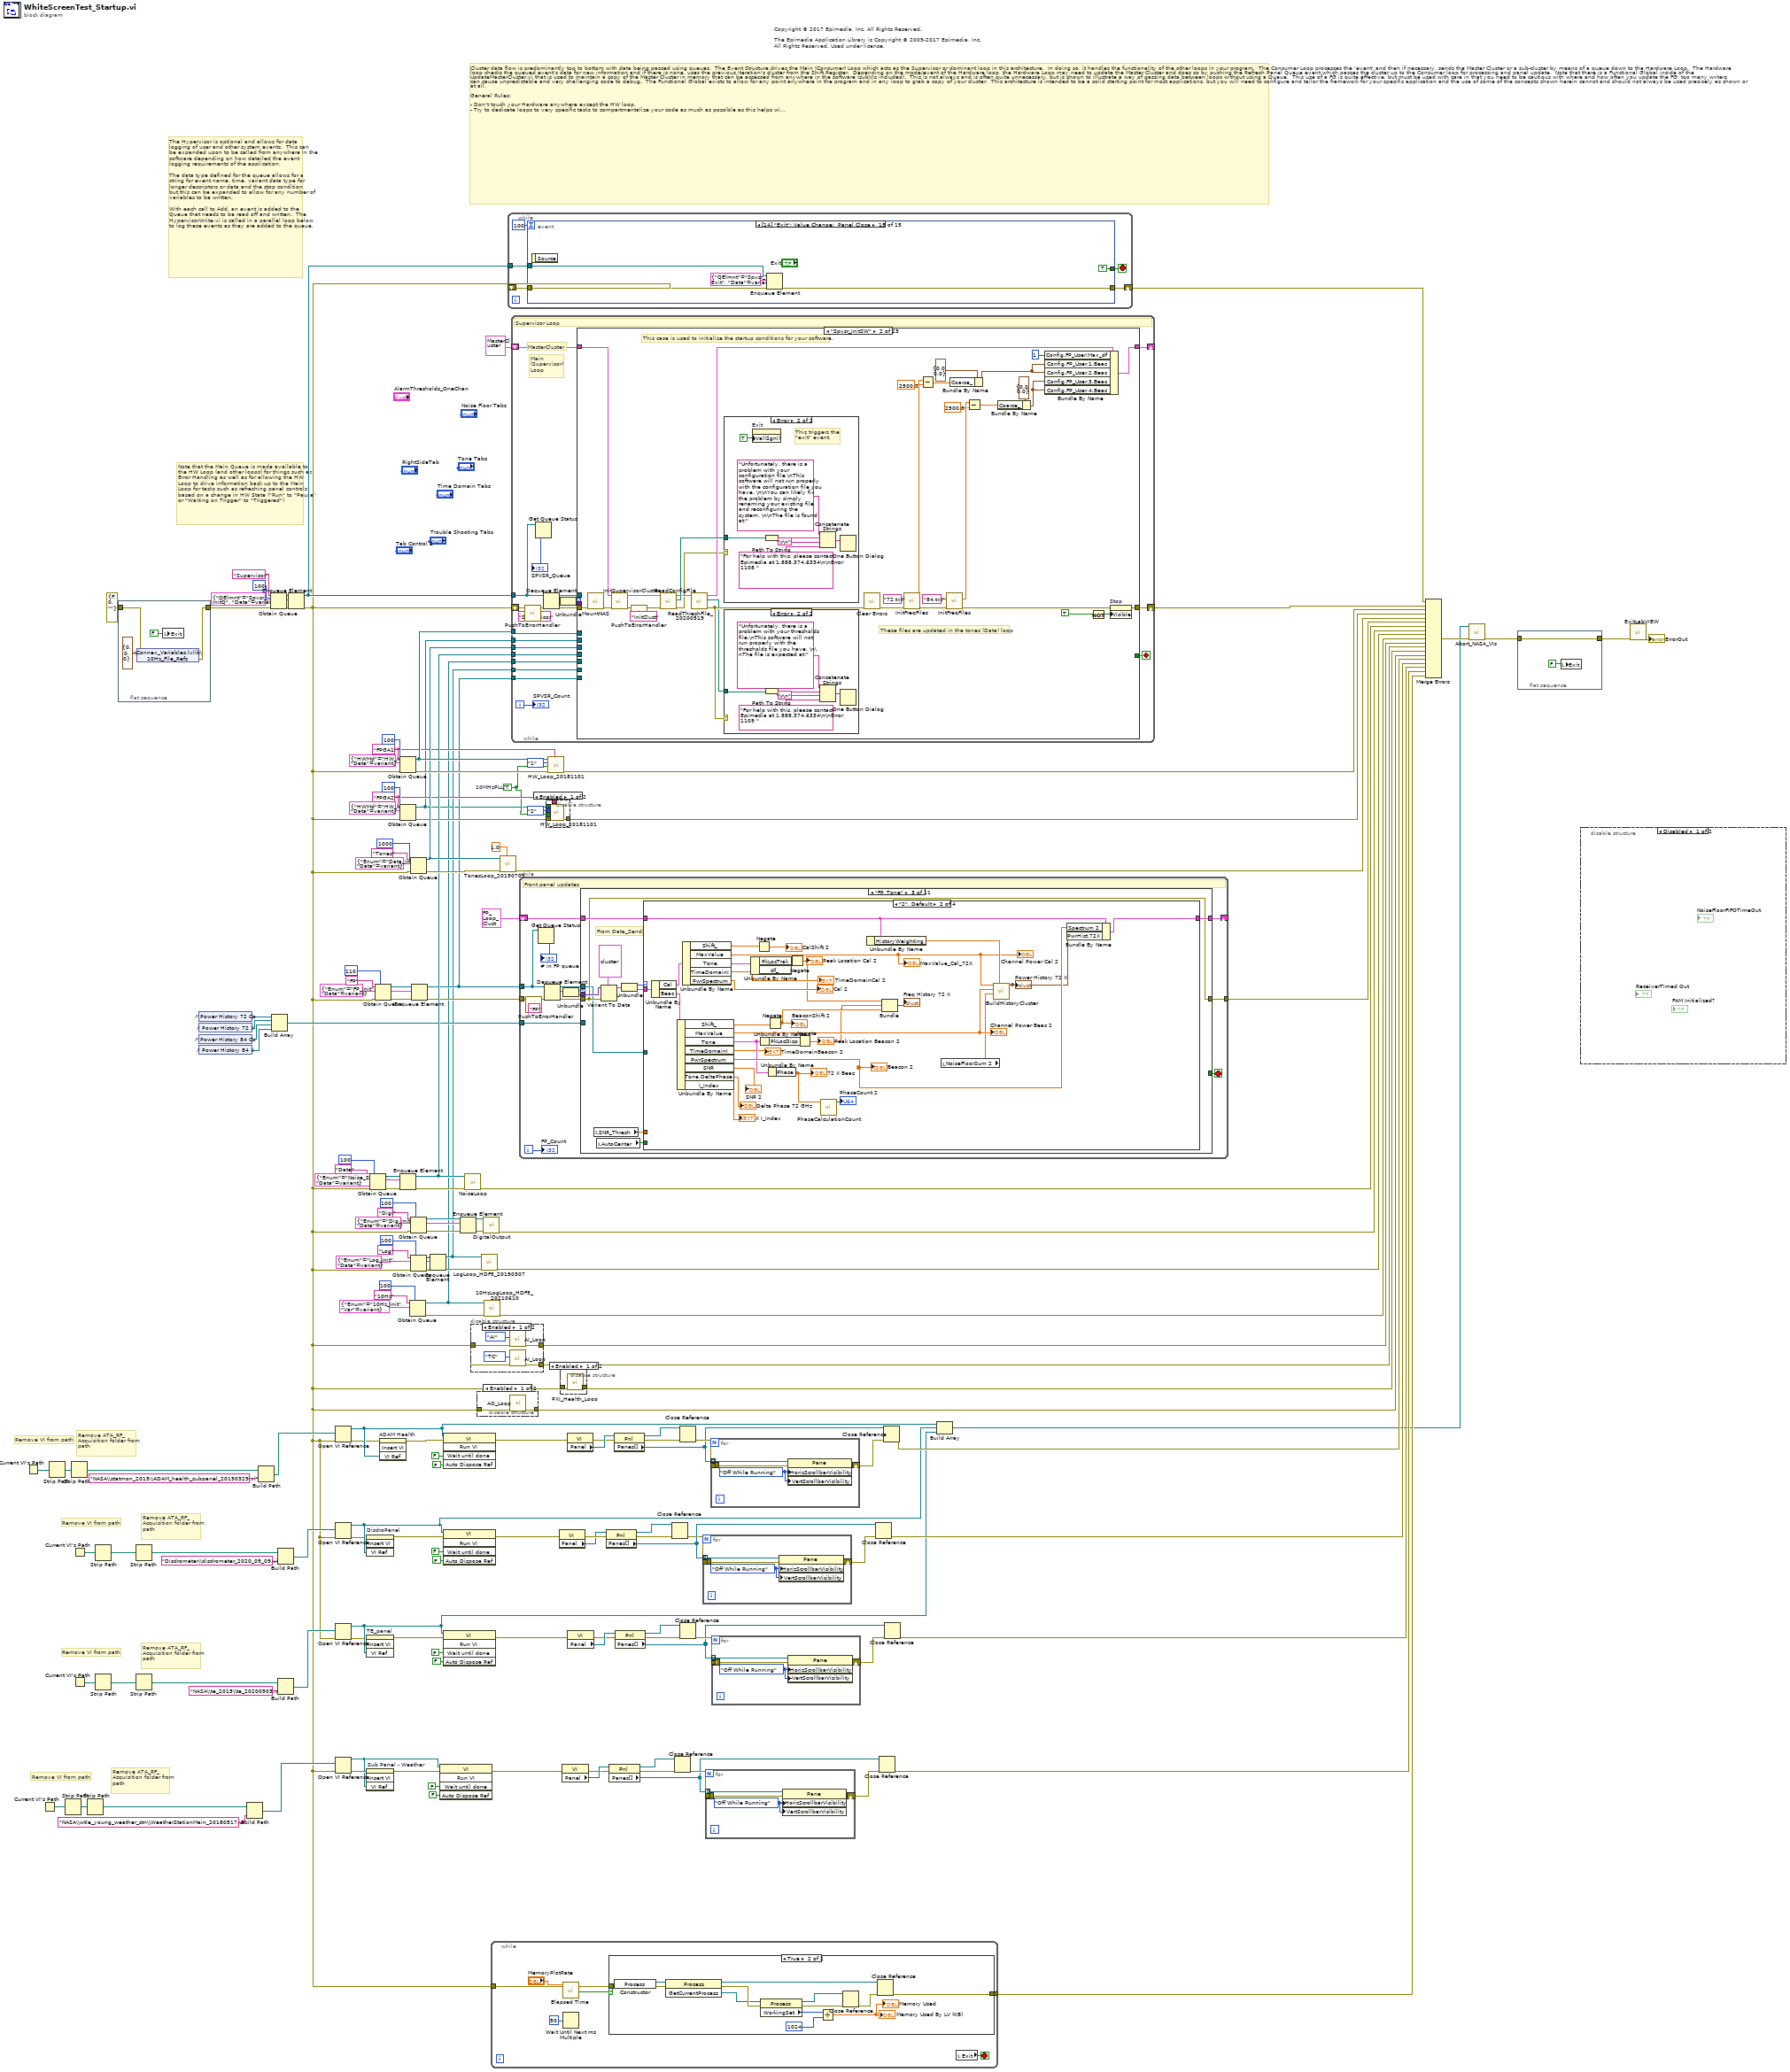
[diagram p0: block diagram]
diagram:
  w64 = TRUE  # 10MHzPLL?
  w114 = "FPGA2" ("name (unnamed)")
  w97 = cluster{"Enum":T28, "Data":variant} {"Enum"=enum."FP_Init", "Data"=variant}
  w124 = cluster{"Enum":T29, "Data":variant} {"Enum"=enum."Dig_Init", "Data"=variant}
  w65 = cluster{"Enum":T30, "Data":variant} {"Enum"=enum."Log_Init", "Data"=variant}
  w118 = cluster{"Enum":T31, "Data":variant} {"Enum"=enum."Noise_Startup", "Data"=variant}
